vi "test_libssh2_channel_flush_stderr.vi"() -> ()   [LabVIEW 2013, in "libssh2_integration_tests.lvlib"]
uses:
  libssh2_integration_tests.lvlib
  <vilib>/addons/_JKI Toolkits/Caraya/classes/Test/Test.lvclass
  libssh2/libssh2.lvlib
  <vilib>/addons/_JKI Toolkits/Caraya/classes/Assert/Assert.lvclass
panel:
  out "error out":errorcluster
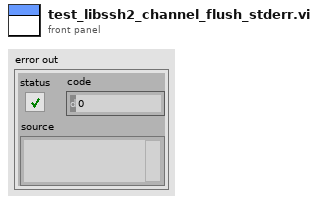
[diagram p1: front panel]
types:
  T1 = typedef "libssh2.lvlib/Session Refnum.ctl" = refnum<k1>
  T2 = typedef "libssh2.lvlib/Channel Refnum.ctl" = refnum<k1>
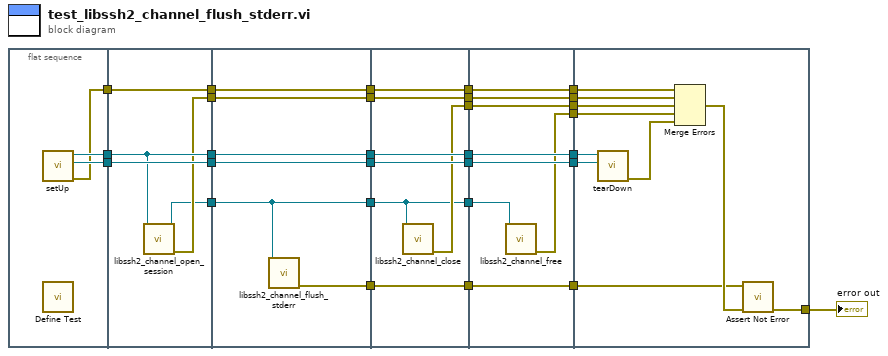
[diagram p0: block diagram]
diagram:
  n1 = flat-sequence {
    tunnel: [w32] -> w29
    tunnel: [w31] -> w28
    tunnel: [w30] -> w27
    tunnel: w29 -> [w36]
    tunnel: w28 -> [w37]
    tunnel: [w36] -> w11
    tunnel: [w37] -> w10
    tunnel: w27 -> [w35]
    tunnel: [w35] -> w9
    tunnel: [w34] -> w8
    tunnel: [w33] -> w7
    tunnel: w11 -> [w43]
    tunnel: [w43] -> w6
    tunnel: w10 -> [w42]
    tunnel: [w42] -> w5
    tunnel: w9 -> [w41]
    tunnel: [w41] -> w4
    tunnel: w8 -> [w40]
    tunnel: [w40] -> w3
    tunnel: [w39] -> w2
    tunnel: w7 -> [w38]
    tunnel: [w38] -> w1
    tunnel: w6 -> [w50]
    tunnel: w5 -> [w49]
    tunnel: [w50] -> w26
    tunnel: [w49] -> w25
    tunnel: [w44] -> w24
    tunnel: [w48] -> w23
    tunnel: w4 -> [w47]
    tunnel: [w47] -> w22
    tunnel: w3 -> [w46]
    tunnel: [w46] -> w16
    tunnel: w2 -> [w45]
    tunnel: [w45] -> w13
    tunnel: w1 -> [w44]
    tunnel: w26 -> [w58]
    tunnel: w25 -> [w57]
    tunnel: w24 -> [w56]
    tunnel: [w58] -> w21
    tunnel: [w57] -> w20
    tunnel: [w55] -> w19
    tunnel: w23 -> [w54]
    tunnel: [w54] -> w18
    tunnel: w22 -> [w53]
    tunnel: [w53] -> w17
    tunnel: w16 -> [w52]
    tunnel: [w52] -> w15
    tunnel: w13 -> [w51]
    tunnel: [w51] -> w12
    tunnel: w21 -> [w68]
    tunnel: w20 -> [w67]
    tunnel: [w66] -> w14
    tunnel: w19 -> [w64]
    tunnel: w18 -> [w63]
    tunnel: w17 -> [w62]
    tunnel: w15 -> [w60]
    tunnel: w12 -> [w59]
    frame #0 {
      n2 = call "setUp.vi"() -> ("error out"=w30:errorcluster, "connection ID"=w31:refnum<k5>, "session"=w32:T1)  [unwired: 9 in]
      n3 = call <vilib>:"Define Test.vi"() -> ()  [unwired: 10 in, 2 out]
    }
    frame #1 {
      n4 = call "libssh2_channel_open_session.vi"("session"=w36) -> ("error out"=w34:errorcluster, "channel"=w33:T2)  [unwired: 9 in]
    }
    frame #2 {
      n5 = call "libssh2_channel_flush_stderr.vi"("channel"=w38) -> ("error out"=w39:errorcluster)  [unwired: 10 in]
    }
    frame #3 {
      n6 = call "libssh2_channel_close.vi"("channel"=w44) -> ("error out"=w48:errorcluster)  [unwired: 10 in]
    }
    frame #4 {
      n7 = call "libssh2_channel_free.vi"("channel"=w56) -> ("error out"=w55:errorcluster)  [unwired: 10 in]
    }
    frame #5 {
      n8 = call "tearDown.vi"("connection ID"=w67, "session"=w68) -> ("error out"=w65:errorcluster)  [unwired: 9 in]
      n9 = Merge Errors(w62, w60, w63, w64, w65) -> (w61:errorcluster)
      n10 = call <vilib>:"Assert Not Error.vi"("error in (no error)"=w61, "Not Error?"=w59) -> ("error out"=w66:errorcluster)  [unwired: 8 in, 1 out]
    }
  }
  "error out" <- w14
